vi "Tint.vi"(0 "image in":refnum<class "MSC Image.lvclass">, 1 "Tint Type":T1, 5 "error in (no error)":errorcluster) -> (14 "image out":refnum<class "MSC Image.lvclass">, 19 "error out":errorcluster)   [LabVIEW 2014, in "MSC Image.lvclass"]
doc: "Tints the image with selected color."
uses:
  MSC Image.lvclass
  controls/Tint Type.ctl
  MSC Image.lvclass/MSC Image.ctl
  Dependencies/x86/MSC I Process32.dll
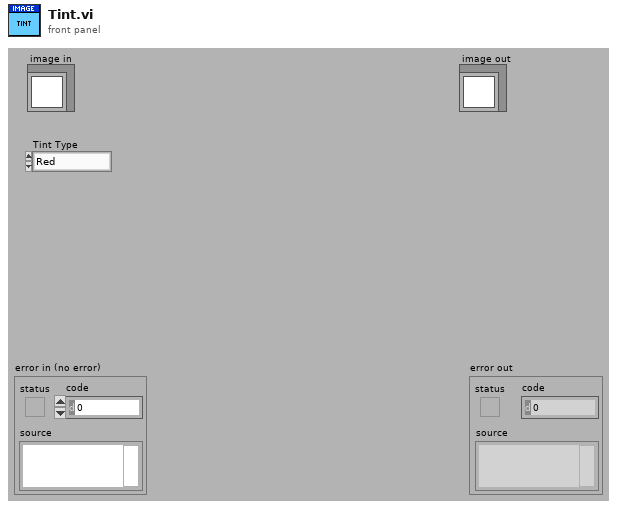
[diagram p1: front panel]
types:
  T1 = typedef "MSC Image.lvclass/Tint Type.ctl" = enum16{"Red", "Green", "Blue", "Cyan", "Magenta", "Yellow"}
  T2 = typedef "Image.ctl" = cluster{"Pointer":u64, "Size":T3, "Image Type":T4, "Time Stamp":timestamp, "Variant":variant}
  T3 = typedef "Size.ctl" = cluster{"Cols":i32, "Rows":i32}
  T4 = typedef "Image Type.ctl" = i32
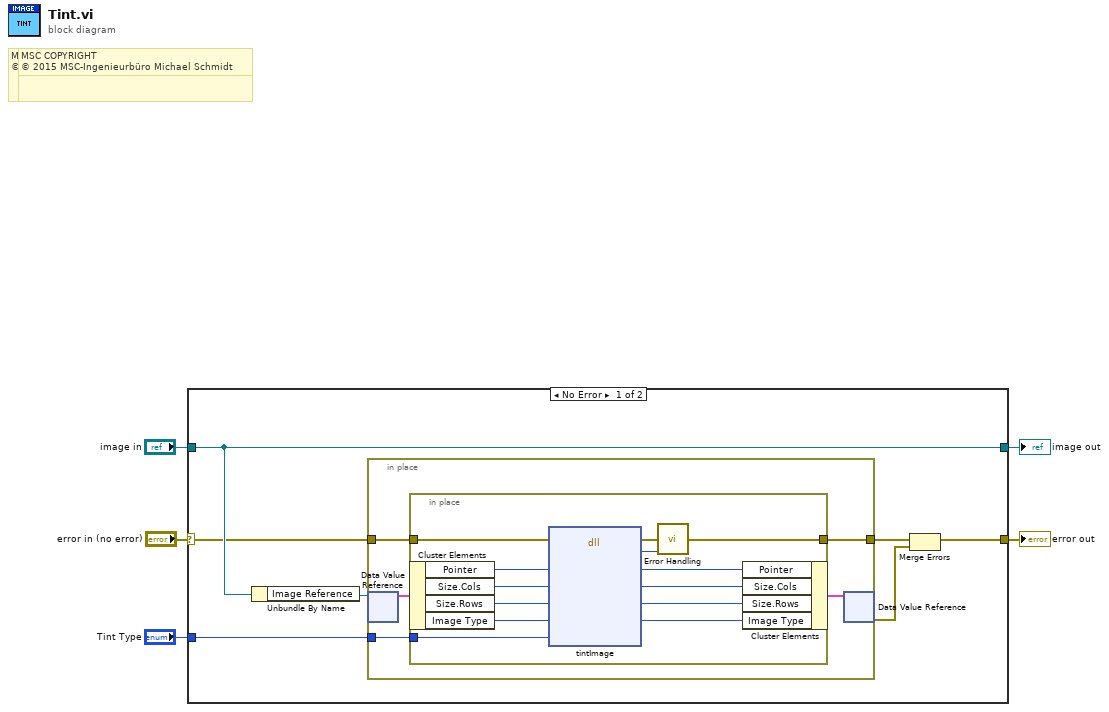
[diagram p0: block diagram]
diagram:
  # "MSC COPYRIGHT\n© 2016 MSC-Ingenieurbüro Michael Schmidt"
  # "MSC COPYRIGHT\n© 2016 MSC-Ingenieurbüro Michael Schmidt"
  # "MSC COPYRIGHT\n© 2015 MSC-Ingenieurbüro Michael Schmidt"
  # "MSC COPYRIGHT\n© 2015 MSC-Ingenieurbüro Michael Schmidt"
  n1 = case shown="No Error" "error in (no error)" {
    selector: "error in (no error)" -> [w8 w32]
    tunnel: [w7 w32] -> w4
    tunnel: [w12 w31] -> w2
    tunnel: "image in" -> [w12 w31]
    tunnel: "Tint Type" -> [w6 _]
    frame No Error {
      n2 = Unbundle By Name(w12) -> ("Image Reference"=w11:refnum<data-value>)
      n3 = in-place {
        in-place-border: w8 -> [w15]
        in-place-border: [w14] -> w10
        in-place-border: w6 -> [w13]
        n4 = in-place-dvr #1(w11) -> (w16:T2)  [unwired: 1 out]
        n5 = in-place {
          in-place-border: w15 -> [w29]
          in-place-border: [w30] -> w14
          in-place-border: w13 -> [w18]
          n6 = in-place-cluster #2(w16) -> ("Pointer"=w26:u64, "Size.Cols"=w25:i32, "Size.Rows"=w24:i32, "Image Type"=w23:T4)
          n7 = dll-call lib="C:/Users/MSC/LabVIEW Projekte/LV 2014/MSC I-Process/user.lib/MSC-I Process/Dependencies/x86/MSC I Process*.dll" fn="tintImage"(error in=w29, "pointer"=w26, "cols"=w25, "rows"=w24, "type"=w23, "tintType"=w18) -> (error out=w28:errorcluster, "error"=w27:i32, "pointer"=w19:u64, "cols"=w20:i32, "rows"=w21:i32, "type"=w22:i32)  [unwired: 3 in, 1 out]
          n8 = call "Error Handling.vi"("error in (no error)"=w28, "return type"=w27) -> ("error out"=w30:errorcluster)  [unwired: 12 in, 1 out]
          n9 = in-place-cluster #2("Pointer"=w19, "Size.Cols"=w20, "Size.Rows"=w21, "Image Type"=w22) -> (w17:T2)
        }
        n10 = in-place-dvr #1(w17) -> (w9:errorcluster)  [unwired: 1 out]
      }
      n11 = Merge Errors(w10, w9) -> (w7:errorcluster)
    }
    frame Error {
    }
  }
  "error out" <- w4
  "image out" <- w2
